vi "KI.vi"() -> ()   [LabVIEW 2020]
uses:
  <vilib>/Utility/error.llb/DialogType.ctl
  <vilib>/DAQmx/read.llb/DAQmx Read (Analog 1D Wfm NChan NSamp).vi
  <vilib>/DAQmx/create/channels.llb/DAQmx Create Channel (AI-Voltage-Basic).vi
  <vilib>/DAQmx/configure/timing.llb/DAQmx Timing (Sample Clock).vi
  <vilib>/DAQmx/miscellaneous.llb/DAQmx Fill In Error Info.vi
  <vilib>/measure/madcrms.llb/Basic Averaged DC-RMS for 1 Chan.vi
  <resource>/objmgr/daqmx.rc
  <vilib>/measure/NI_MAPro.lvlib
panel:
  out "data":string
  out "KI":dbl
  out "I_Amp [A]":dbl
  out "V_DAQ [V]":dbl
  in  "%Reading V":dbl
  in  "%Range V":dbl
  in  "Range V":dbl
  out "Emax I [A]":dbl
  out "U(I) (type B)":dbl
  out "U(D) (type A)":dbl
  out "Uc":dbl
  out "Waveform Graph":waveform(dbl)[](graph)
  in  "Command":string
  in  "address GPIB":string
  out "Actual sample clk  rate":dbl
  in  "sample clock source":tag
  in  "sample rate":dbl=1000.0 format="%0.2f"
  in  "n of samples":i32=1000
  in  "physical channel":tag
  in  "input terminal configuration":i32(ring)=-1 items=["Default"=-1, "RSE"=10083, "NRSE"=10078, "Differential"=10106, "Pseudodifferential"=12529]
  in  "Min V":dbl=-5.0 format="%0.2f"
  in  "Max V":dbl=5.0 format="%0.2f"
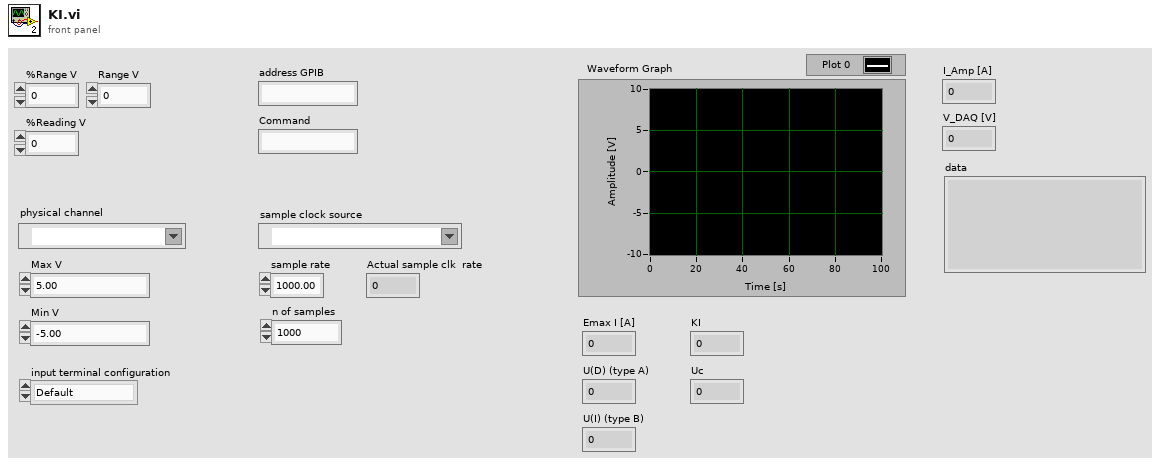
[diagram p1: front panel]
types:
  T1 = typedef "DialogType.ctl" = u16
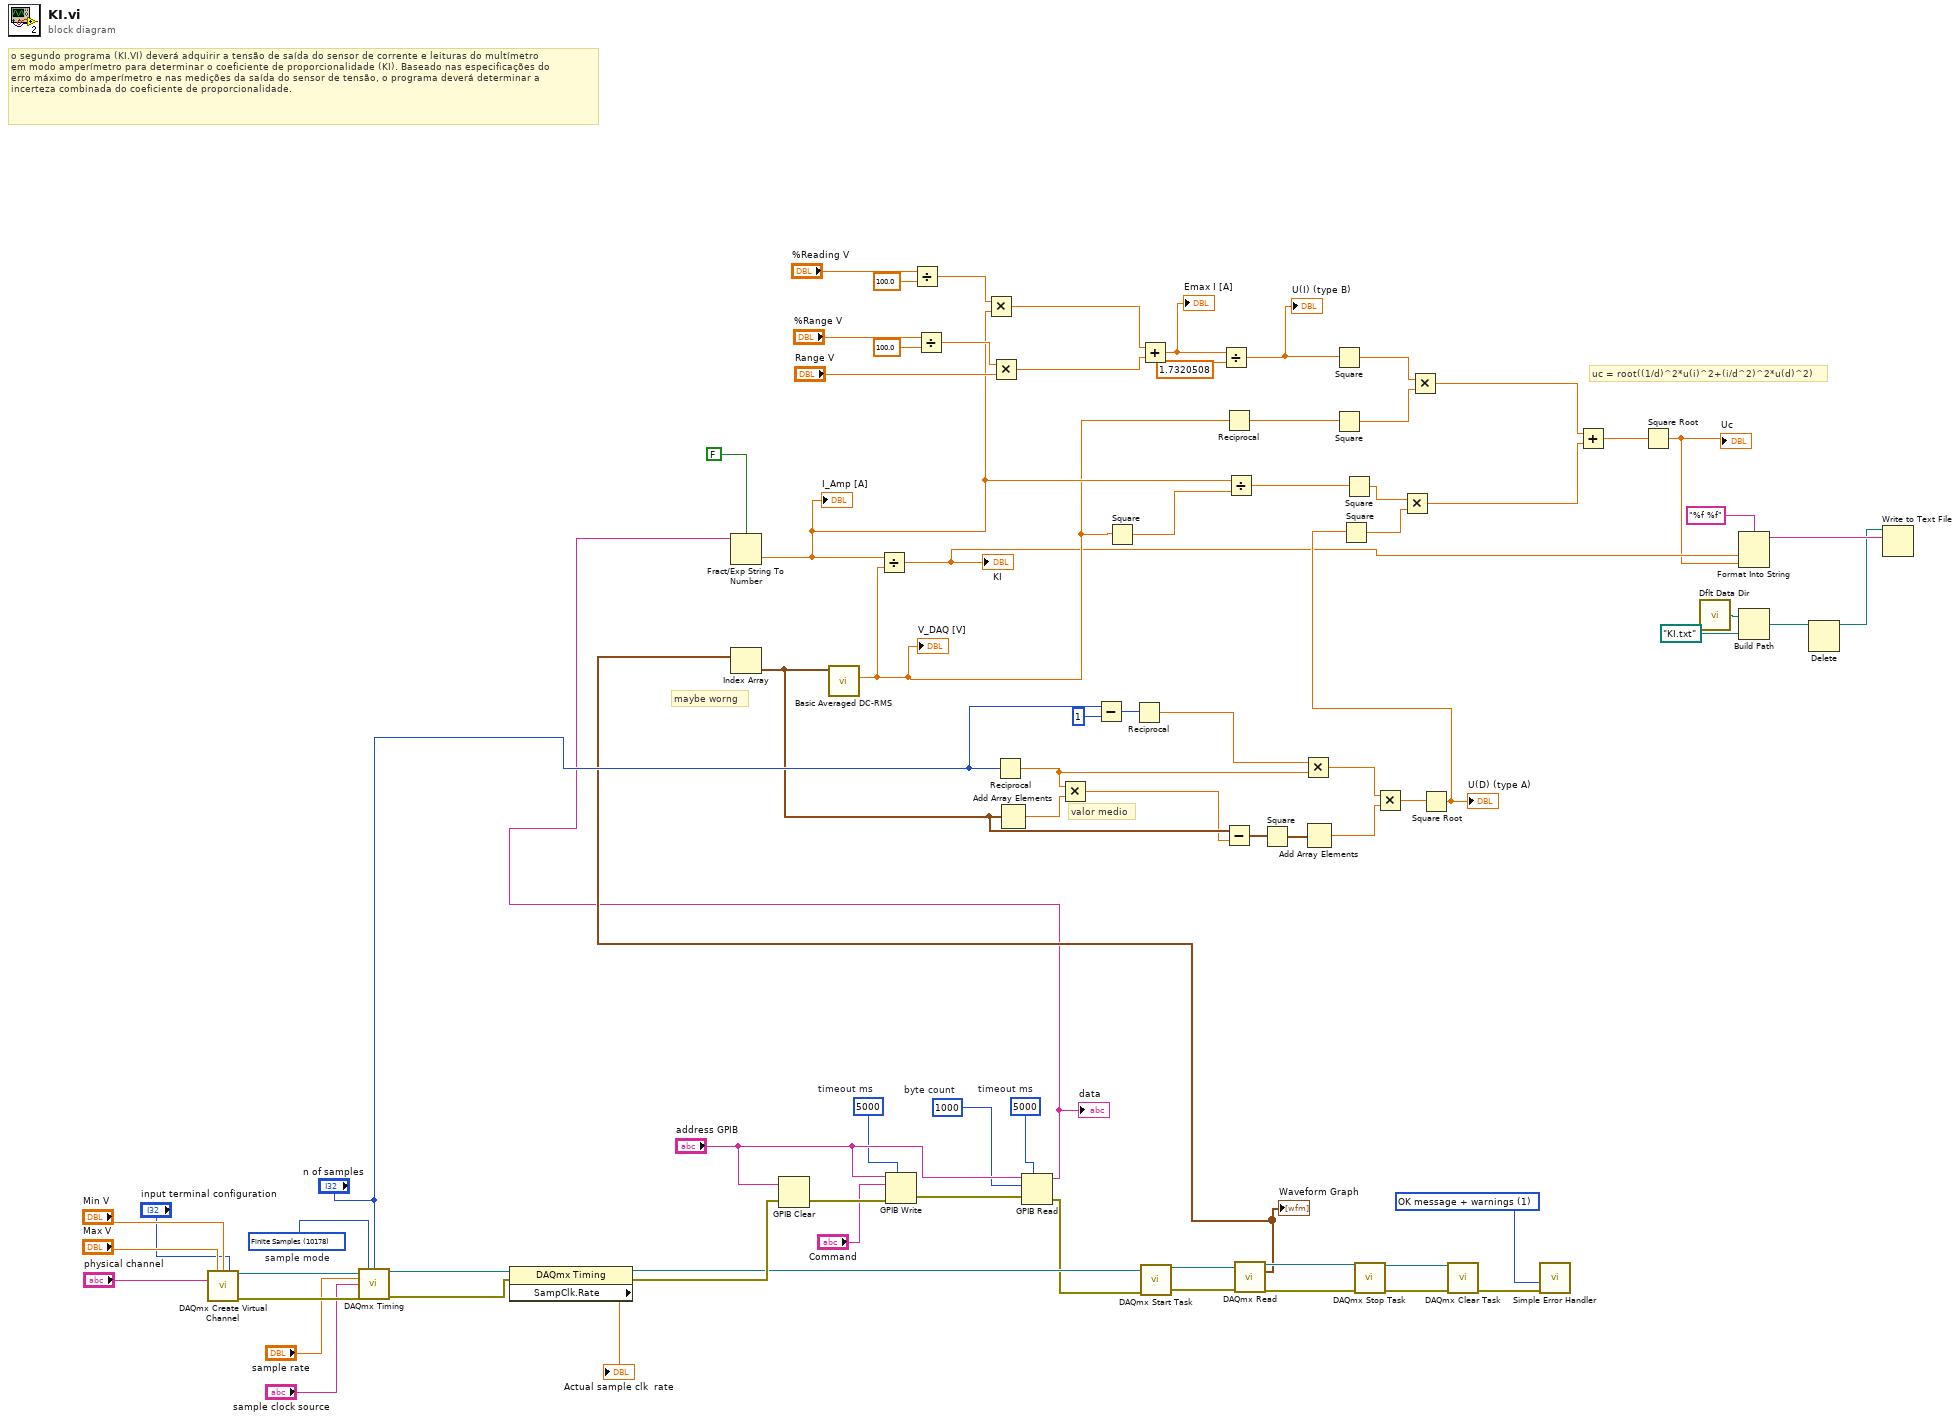
[diagram p0: block diagram]
diagram:
  w61 = 5000  # timeout ms
  w62 = 1000  # byte count
  w63 = 5000  # timeout ms
  w51 = T1 1 items=["no dialog", "OK message + warnings", "OK message", "continue or stop message", "continue/stop + warnings"] ("type of dialog (OK msg:1)")
  w71 = 10178 items=["Finite Samples"=10178, "Continuous Samples"=10123, "Hardware Timed Single Point"=12522]  # sample mode
  # "valor medio"
  # "maybe worng"
  # "uc = root((1/d)^2*u(i)^2+(i/d^2)^2*u(d)^2)"
  # "o segundo programa (KI.VI) deverá adquirir a tensão de saída do sensor de corrente e leituras do multímetro\nem modo amperímetro para determinar o coeficiente de proporcionalidade (KI). Baseado nas especificações do\nerro máximo do amperímetro e nas medições da saída do sensor de tensão, o programa deverá determinar a\nincerteza combinada do coeficiente de proporcionalidade."
  n1 = call-poly <vilib>:"DAQmx Create Virtual Channel.vi"("maximum value"="Max V", "minimum value"="Min V", "input terminal configuration"="input terminal configuration", "physical channels"="physical channel") -> ("task out"=w79:refnum<k21>, "error out"=w78:errorcluster)  [unwired: 10 in]
  n2 = call-poly <vilib>:"DAQmx Timing.vi"("task/channels in"=w79, "sample mode"=w71, "samples per channel"="n of samples", "rate"="sample rate", "source"="sample clock source", "error in"=w78) -> ("task out"=w76:refnum<k21>, "error out"=w77:errorcluster)  [unwired: 8 in]
  n3 = property class="DAQmx Timing"(reference=w76, error in=w77) -> (reference out=w60:refnum<k21>, error out=w68:errorcluster, "SampClk.Rate"=→"Actual sample clk  rate":dbl)
  n4 = GPIB Clear(2:w68, 3:"address GPIB") -> (0:w67:errorcluster)  [unwired: 1 out]
  n5 = GPIB Write(0:"address GPIB", 1:"Command", 3:w67, 4:w63) -> (6:w66:errorcluster)  [unwired: 1 in, 1 out]
  n6 = Divide(x="%Reading V", y=100.0) -> (x/y=w42:dbl)
  n7 = Divide(x="%Range V", y=100.0) -> (x/y=w41:dbl)
  n8 = Multiply(x=w41, y="Range V") -> (x*y=w38:dbl)
  n9 = Reciprocal(x="n of samples") -> (1/x=w27:dbl)
  n10 = GPIB Read(0:"address GPIB", 1:w62, 3:w66, 4:w61) -> (5:w47:string, 7:w59:errorcluster)  [unwired: 1 in, 1 out]
  "data" <- w47
  n11 = Fract/Exp String To Number(use system decimal point (T)=FALSE, string=w47) -> (number=w17:dbl)  [unwired: 2 in, 1 out]
  "I_Amp [A]" <- w17
  n12 = Multiply(x=w42, y=w17) -> (x*y=w39:dbl)
  n13 = Subtract(x="n of samples", y=1) -> (x-y=w28:i32)
  n14 = Reciprocal(x=w28) -> (1/x=w26:dbl)
  n15 = Add(x=w39, y=w38) -> (x+y=w37:dbl)
  "Emax I [A]" <- w37
  n16 = call <vilib>:"DAQmx Start Task.vi"("task/channels in"=w60, "error in"=w59) -> ("task out"=w58:refnum<k21>, "error out"=w53:errorcluster)  [unwired: 12 in]
  n17 = Divide(x=w37, y=1.7320508) -> (x/y=w34:dbl)
  "U(I) (type B)" <- w34
  n18 = call-poly <vilib>:"DAQmx Read.vi"("task/channels in"=w58, "error in"=w53) -> ("task out"=w57:refnum<k21>, "data"=w48:waveform(dbl)[], "error out"=w54:errorcluster)  [unwired: 11 in]
  "Waveform Graph" <- w48
  n19 = Index Array(array=w48) -> (element=w25:waveform(dbl))  [unwired: 1 in]
  n20 = call-poly <vilib>:"Basic Averaged DC-RMS.vi"("signal in"=w25) -> ("RMS value"=w16:dbl)  [unwired: 7 in, 3 out]
  "V_DAQ [V]" <- w16
  n21 = Divide(x=w17, y=w16) -> (x/y=w3:dbl)
  "KI" <- w3
  n22 = Add Array Elements(numeric array=w25) -> (sum=w30:dbl)
  n23 = Multiply(x=w27, y=w30) -> (x*y=w24:dbl)
  n24 = Square(x=w16) -> (x^2=w15:dbl)
  n25 = Reciprocal(x=w16) -> (1/x=w33:dbl)
  n26 = Subtract(x=w25, y=w24) -> (x-y=w23:waveform(dbl))
  n27 = Divide(x=w17, y=w15) -> (x/y=w14:dbl)
  n28 = Square(x=w23) -> (x^2=w22:waveform(dbl))
  n29 = Multiply(x=w26, y=w27) -> (x*y=w21:dbl)
  n30 = Add Array Elements(numeric array=w22) -> (sum=w20:dbl)
  n31 = Square(x=w34) -> (x^2=w32:dbl)
  n32 = Square(x=w33) -> (x^2=w31:dbl)
  n33 = Square(x=w14) -> (x^2=w13:dbl)
  n34 = call <vilib>:"DAQmx Stop Task.vi"("task/channels in"=w57, "error in"=w54) -> ("task out"=w56:refnum<k21>, "error out"=w55:errorcluster)  [unwired: 12 in]
  n35 = Multiply(x=w21, y=w20) -> (x*y=w19:dbl)
  n36 = Multiply(x=w32, y=w31) -> (x*y=w11:dbl)
  n37 = Square Root(x=w19) -> (sqrt(x)=w18:dbl)
  "U(D) (type A)" <- w18
  n38 = Square(x=w18) -> (x^2=w12:dbl)
  n39 = Multiply(x=w13, y=w12) -> (x*y=w10:dbl)
  n40 = call <vilib>:"DAQmx Clear Task.vi"("task in"=w56, "error in"=w55) -> ("error out"=w52:errorcluster)  [unwired: 13 in]
  n41 = call <vilib>:"Simple Error Handler.vi"("type of dialog (OK msg:1)"=w51, "error in (no error)"=w52) -> ()  [unwired: 3 in, 5 out]
  n42 = Add(x=w11, y=w10) -> (x+y=w9:dbl)
  n43 = Square Root(x=w9) -> (sqrt(x)=w2:dbl)
  "Uc" <- w2
  n44 = call <vilib>:"Dflt Data Dir.vi"() -> ("App:Default Data Directory"=w6:path)
  n45 = Format Into String(format string="%f %f", w3, w2) -> (resulting string=w7:string)  [unwired: 2 in, 1 out]
  n46 = Build Path(base path=w6, name or relative path=path "KI.txt" ("base path")) -> (appended path=w5:path)
  n47 = Delete(path (use dialog)=w5) -> (deleted path=w4:path)  [unwired: 4 in, 2 out]
  n48 = Write to Text File(file (use dialog)=w4, text=w7) -> ()  [unwired: 2 in, 3 out]
